vi "sInitialization.vi"(8 "UTC format":bool=TRUE, 9 "XOFF Character":u8=19 format="%.0x", 10 "XON Character":u8=17 format="%.0x", 11 "VISA resource name":refnum<visa-resource-name>="COM5") -> (0 "error IO":errorcluster, 3 "VISA resource name out":refnum<visa-resource-name>, 5 "Slow Cluster":T1)   [LabVIEW 2012]
uses:
  <vilib>/Instr/_visa.llb/VISA Configure Serial Port (Instr).vi
panel:
  out "Datanames":string[](array[string])
  out "Description":string[](array[string])
  out "Up bound":i32[](array[numeric])
  out "Low bound":i32[](array[numeric])
  out "Stopped":bool
  out "array of datanames":string[](array[string])
  out "array of datanames 2":string[](array[string])
  out "Arduino needs to be reinitialized":bool
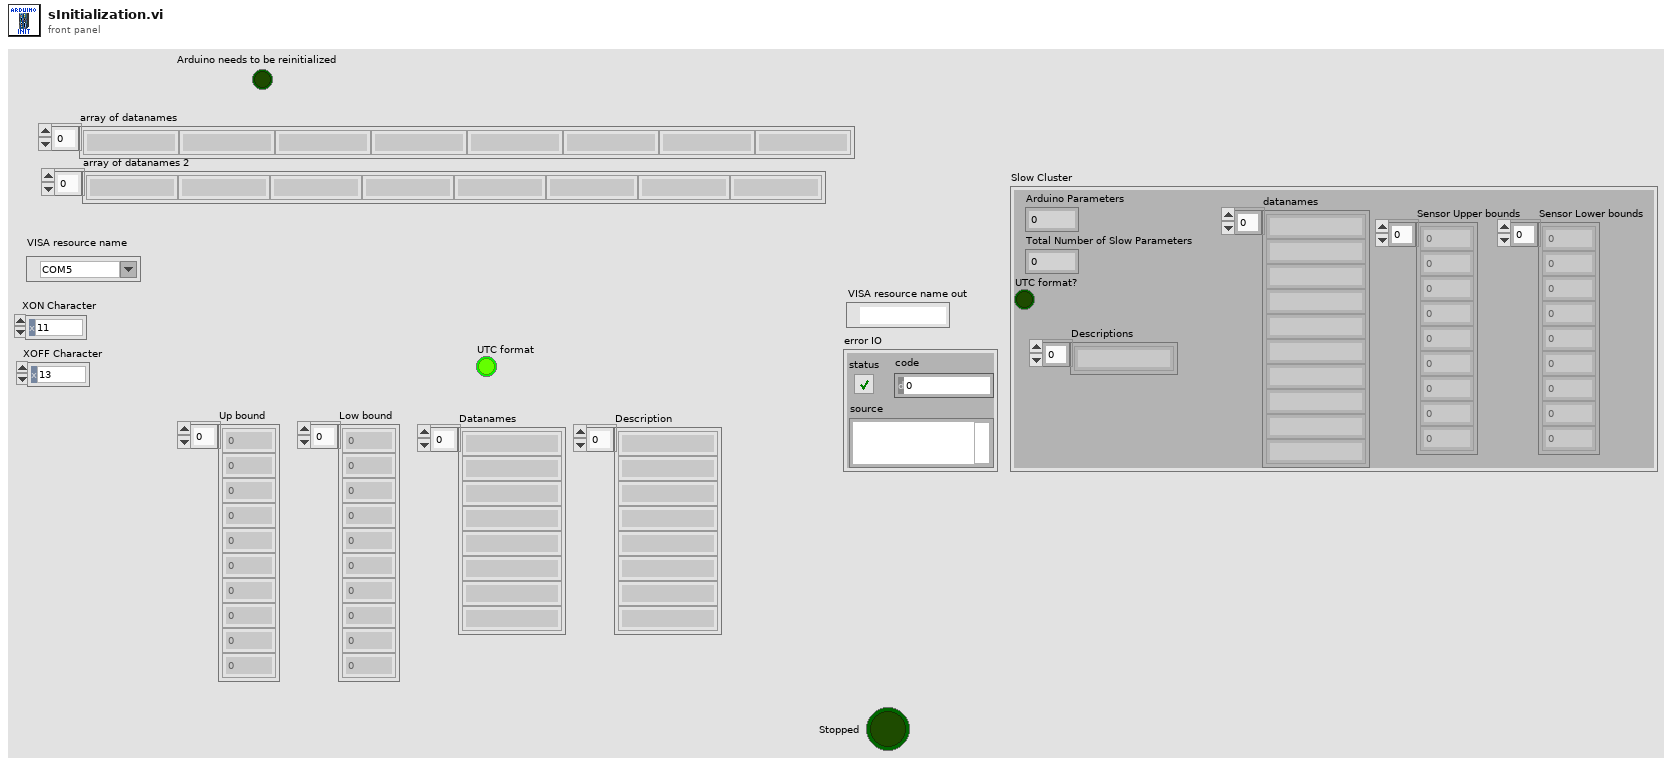
[diagram p1: front panel]
types:
  T1 = cluster{"Arduino Parameters":dbl, "Total Number of Slow Parameters":i32, "UTC format?":bool, "Sensor Upper bounds":i32[], "Sensor Lower bounds":i32[], "Descriptions":string[], "datanames":string[]}
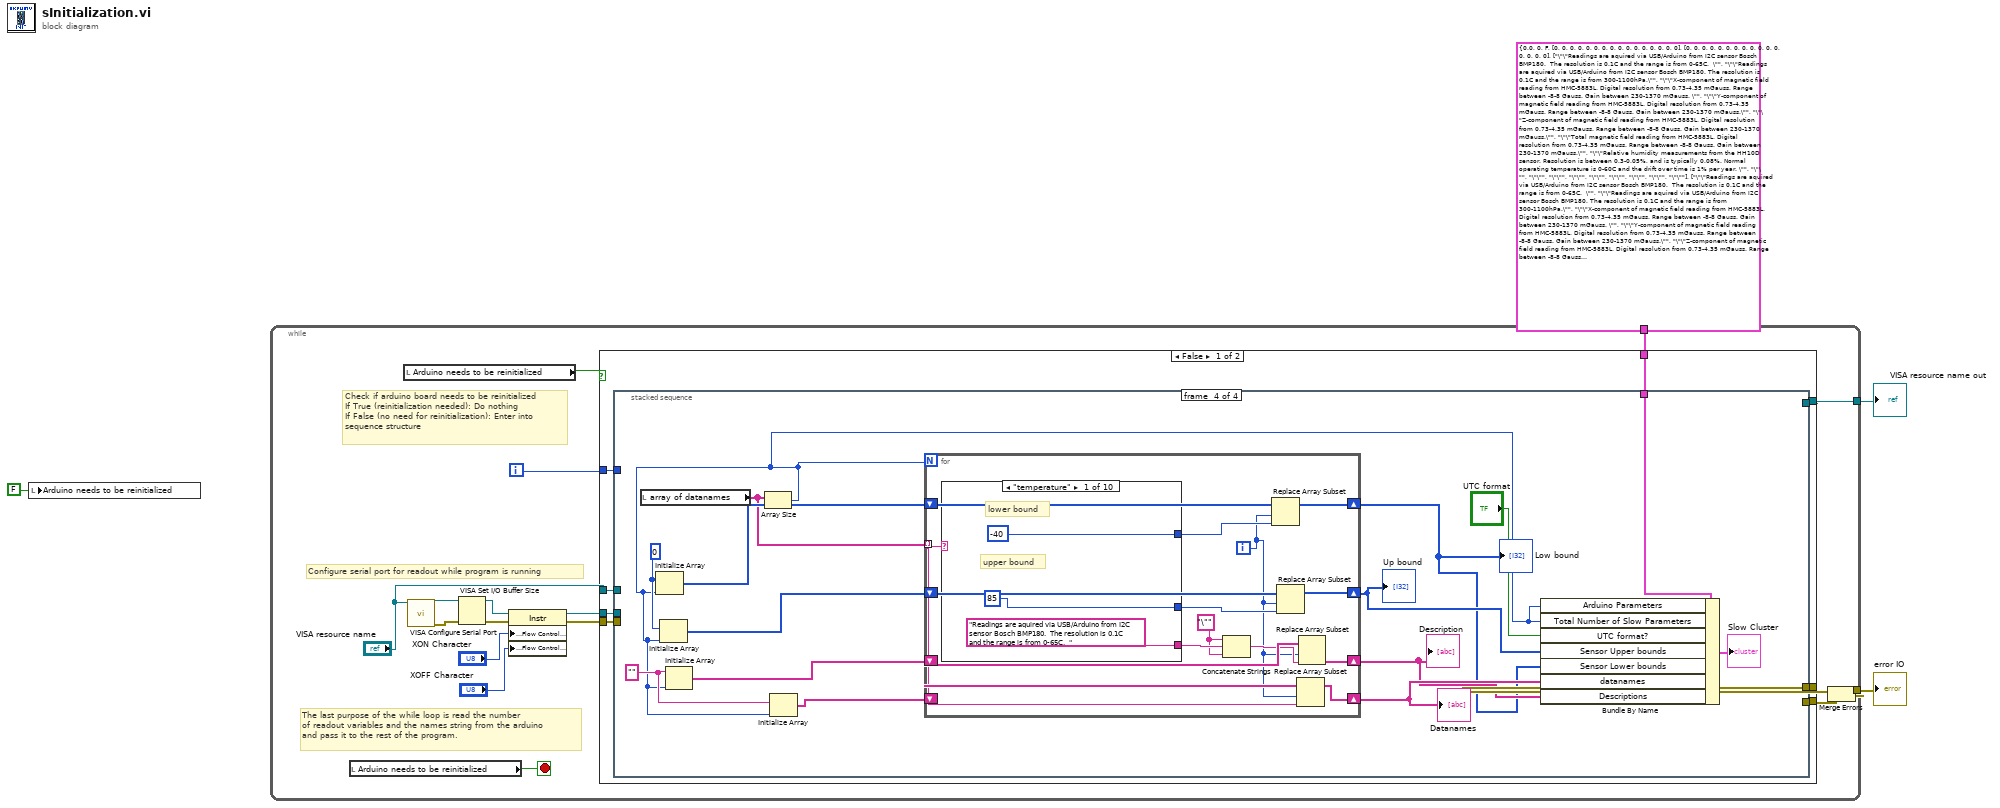
[diagram p0: block diagram]
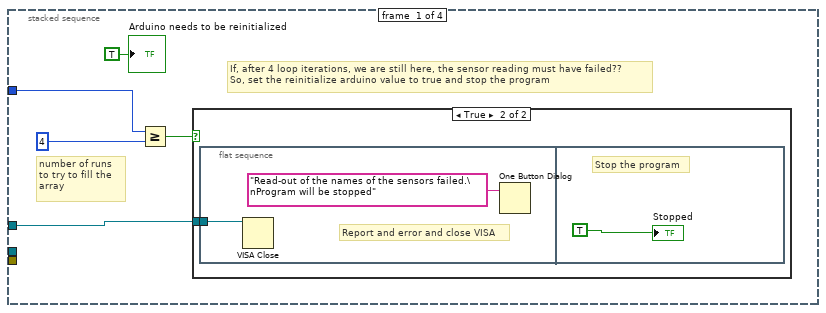
[diagram p2: hidden frame]
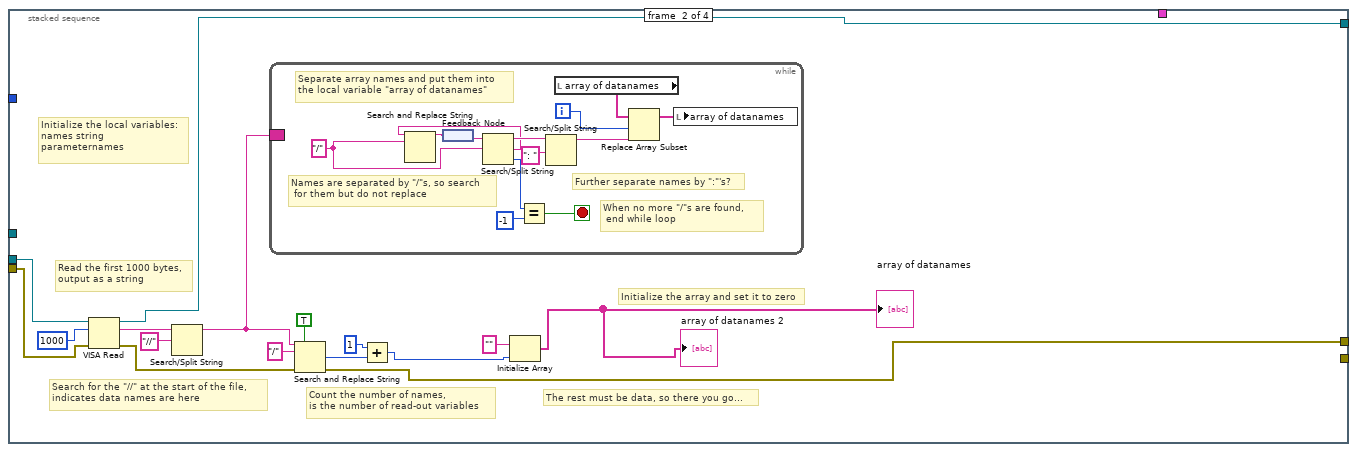
[diagram p4: hidden frame]
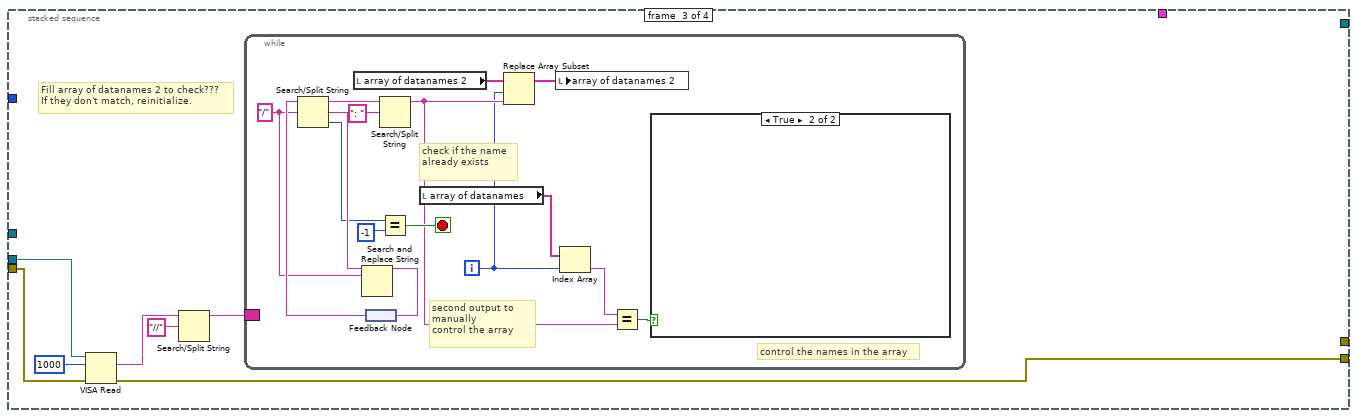
[diagram p5: hidden frame]
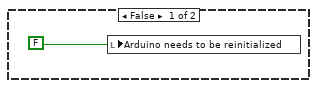
[diagram p6: hidden frame]
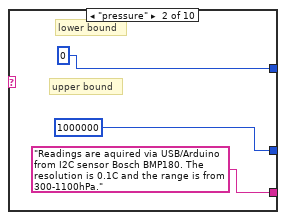
[diagram p7: hidden frame]
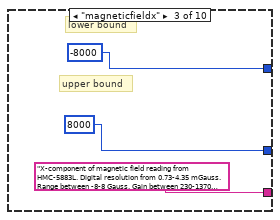
[diagram p8: hidden frame]
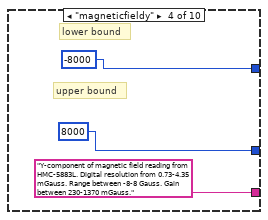
[diagram p9: hidden frame]
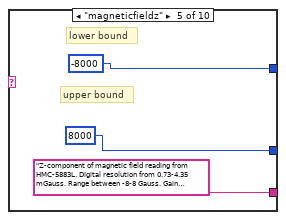
[diagram p10: hidden frame]
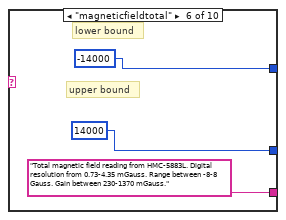
[diagram p11: hidden frame]
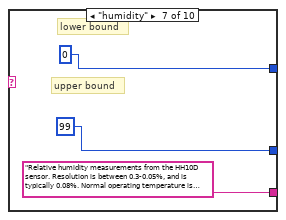
[diagram p12: hidden frame]
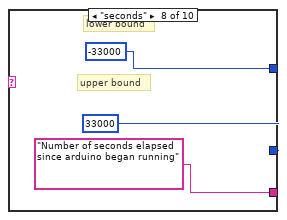
[diagram p13: hidden frame]
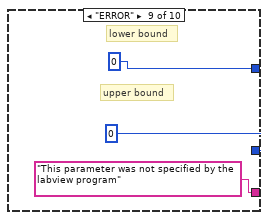
[diagram p14: hidden frame]
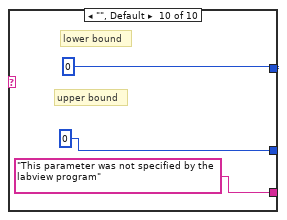
[diagram p15: hidden frame]
diagram:
  n1 = local write "Arduino needs to be reinitialized"(FALSE ("Arduino needs to be reinitialized")) -> ()
  n2 = while {
    tunnel: [w15] -> w4
    tunnel: [w14] -> w3
    tunnel: T1 {"Arduino Parameters"=0.0, "Total Number of Slow Parameters"=0, "UTC format?"=FALSE, "Sensor Upper bounds"=[0, 0, 0, 0, 0, 0, 0, 0, 0, 0, 0, 0, 0, 0, 0, 0], "Sensor Lower bounds"=[0, 0, 0, 0, 0, 0, 0, 0, 0, 0, 0, 0, 0, 0, 0, 0], "Descriptions"=["\"\"Readings are aquired via USB/Arduino from I2C sensor Bosch BMP180.  The resolution is 0.1C and the range is from 0-65C.  \"", "\"\"Readings are aquired via USB/Arduino from I2C sensor Bosch BMP180. The resolution is 0.1C and the range is from 300-1100hPa.\"", "\"\"X-component of magnetic field reading from HMC-5883L. Digital resolution from 0.73-4.35 mGauss. Range between -8-8 Gauss. Gain between 230-1370 mGauss. \"", "\"\"Y-component of magnetic field reading from HMC-5883L. Digital resolution from 0.73-4.35 mGauss. Range between -8-8 Gauss. Gain between 230-1370 mGauss.\"", "\"\"Z-component of magnetic field reading from HMC-5883L. Digital resolution from 0.73-4.35 mGauss. Range between -8-8 Gauss. Gain between 230-1370 mGauss.\"", "\"\"Total magnetic field reading from HMC-5883L. Digital resolution from 0.73-4.35 mGauss. Range between -8-8 Gauss. Gain between 230-1370 mGauss.\"", "\"\"Relative humidity measurements from the HH10D sensor. Resolution is between 0.3-0.05%, and is typically 0.08%. Normal operating temperature is 0-60C and the drift over time is 1% per year. \"", "\"\"", "\"\"", "\"\"", "\"\"", "\"\"", "\"\"", "\"\"", "\"\"", "\"\""], "datanames"=["\"\"Readings are aquired via USB/Arduino from I2C sensor Bosch BMP180.  The resolution is 0.1C and the range is from 0-65C.  \"", "\"\"Readings are aquired via USB/Arduino from I2C sensor Bosch BMP180. The resolution is 0.1C and the range is from 300-1100hPa.\"", "\"\"X-component of magnetic field reading from HMC-5883L. Digital resolution from 0.73-4.35 mGauss. Range between -8-8 Gauss. Gain between 230-1370 mGauss. \"", "\"\"Y-component of magnetic field reading from HMC-5883L. Digital resolution from 0.73-4.35 mGauss. Range between -8-8 Gauss. Gain between 230-1370 mGauss.\"", "\"\"Z-component of magnetic field reading from HMC-5883L. Digital resolution from 0.73-4.35 mGauss. Range between -8-8 Gauss. Gain between 230-1370 mGauss.\"", "\"\"Total magnetic field reading from HMC-5883L. Digital resolution from 0.73-4.35 mGauss. Range between -8-8 Gauss. Gain between 230-1370 mGauss.\"", "\"\"Relative humidity measurements from the HH10D sensor. Resolution is between 0.3-0.05%, and is typically 0.08%. Normal operating temperature is 0-60C and the drift over time is 1% per year. \"", "\"\"", "\"\"", "\"\"", "\"\"", "\"\"", "\"\"", "\"\"", "\"\"", "\"\""]} ("Cluster") -> [w5]
    i -> [w12]
    stop <- w10 stop-if-true
    # "The last purpose of the while loop is read the number \nof readout variables and the names string from the arduino\nand pass it to the rest of the program."
    # "Check if arduino board needs to be reinitialized\nIf True (reinitialization needed): Do nothing\nIf False (no need for reinitialization): Enter into \nsequence structure"
    # "Configure serial port for readout while program is running"
    n3 = local read "Arduino needs to be reinitialized"() -> (w10:bool)
    n4 = local read "Arduino needs to be reinitialized"() -> (w9:bool)
    n5 = call-poly "VISA Configure Serial Port"("VISA resource name"="VISA resource name") -> ("VISA resource name out"=w17:refnum<visa-resource-name>, "error out"=w16:errorcluster)  [unwired: 9 in, 4 out]
    n6 = VISA Set I/O Buffer Size(VISA resource name=w17, error in (no error)=w16) -> (VISA resource name out=w21:refnum<visa-resource-name>, error out=w20:errorcluster)  [unwired: 2 in]
    n7 = property class="Instr"(reference=w21, error in=w20, "Serial Settings:Flow Control XON Character"="XON Character", "Serial Settings:Flow Control XOFF Character"="XOFF Character") -> (reference out=w13:refnum<visa-resource-name>, error out=w8:errorcluster)
    n8 = case shown="False" w9 {
      tunnel: [w29 w152] -> w15
      tunnel: w13 -> [w28 w152]
      tunnel: w12 -> [w27 _]
      tunnel: "VISA resource name" -> [w26 _]
      tunnel: w8 -> [w25 _]
      tunnel: [w24 _] -> w7
      tunnel: [w23 _] -> w6
      tunnel: w5 -> [w22 _]
      frame False {
        n9 = stacked-sequence {
          tunnel: [_ w51 _ _] -> w29
          tunnel: w28 -> [_ w54 w71 _]
          tunnel: w27 -> [w34 _ _ _]
          tunnel: w26 -> [w31 _ _ _]
          tunnel: w25 -> [_ w52 w69 _]
          tunnel: [_ w41 _ _] -> w24
          tunnel: [_ _ w68 _] -> w23
          tunnel: w22 -> [_ _ _ w93]
          frame #0 {
            # "If, after 4 loop iterations, we are still here, the sensor reading must have failed??  \nSo, set the reinitialize arduino value to true and stop the program"
            # "number of runs to try to fill the array"
            n10 = Greater Or Equal?(x=w34, y=4) -> (x >= y?=w32:bool)
            n11 = case shown="True" w32 {
              tunnel: w31 -> [_ w35]
              frame False {
              }
              frame True {
                n12 = flat-sequence {
                  tunnel: w35 -> [w36]
                  frame #0 {
                    # "Report and error and close VISA"
                    n13 = VISA Close(VISA resource name=w36) -> ()  [unwired: 1 in, 1 out]
                    n14 = One Button Dialog(message="Read-out of the names of the sensors failed.\nProgram will be stopped") -> ()  [unwired: 1 in, 1 out]
                  }
                  frame #1 {
                    # "Stop the program"
                    "Stopped" <- TRUE ("stop? (T)")
                  }
                }
              }
            }
            "Arduino needs to be reinitialized" <- TRUE ("Arduino needs to be reinitialized")
          }
          frame #1 {
            # "The rest must be data, so there you go..."
            # "Count the number of names, \nis the number of read-out variables"
            # "Search for the \"//\" at the start of the file, \nindicates data names are here"
            # "Initialize the local variables: \nnames string\nparameternames"
            # "Read the first 1000 bytes, \noutput as a string"
            # "Initialize the array and set it to zero"
            n15 = VISA Read(VISA resource name=w54, byte count=u32 1000, error in (no error)=w52) -> (VISA resource name out=w51:refnum<visa-resource-name>, read buffer=w50:string, error out=w42:errorcluster)  [unwired: 1 out]
            n16 = Search/Split String(string=w50, search string/char (-)="//") -> (substring before match=w46:string)  [unwired: 1 in, 2 out]
            n17 = while {
              border: w46 -> [_]
              i -> [w55]
              stop <- w64 stop-if-true
              w60 = "/" ("search string/char (-)")
              # "Further separate names by \":\"'s?"
              # "When no more \"/\"s are found,\n end while loop"
              # "Names are separated by \"/\"s, so search\n for them but do not replace"
              # "Separate array names and put them into \nthe local variable \"array of datanames\""
              n18 = feedback #1() -> (w62:string)
              n19 = Search/Split String(string=w62, search string/char (-)=w60) -> (substring before match=w58:string, match + rest of string=w57:string, offset of match=w59:i32)  [unwired: 1 in]
              n20 = Search and Replace String(input string=w57, search string=w60) -> (result string=w61:string)  [unwired: 6 in, 3 out]
              n21 = feedback-in #1(w61) -> ()
              n22 = Equal?(x=w59, y=-1) -> (x = y?=w64:bool)
              n23 = Search/Split String(string=w58, search string/char (-)=": " ("format string")) -> (substring before match=w56:string)  [unwired: 1 in, 2 out]
              n24 = local read "array of datanames"() -> (w66:string[])
              n25 = Replace Array Subset(array=w66, new element=w56, index=w55) -> (w65:string[])
              n26 = local write "array of datanames"(w65) -> ()
            }
            n27 = Search and Replace String(replace all?=TRUE ("replace all? (F)"), input string=w46, search string="/", error in=w42) -> (number of replacements=w47:i32, error out=w41:errorcluster)  [unwired: 4 in, 2 out]
            n28 = Add(x=1, y=w47) -> (x+y=w39:i32)
            n29 = Initialize Array("", w39) -> (→"array of datanames" →"array of datanames 2":string[])
          }
          frame #2 {
            # "Fill array of datanames 2 to check???\nIf they don't match, reinitialize."
            n30 = VISA Read(VISA resource name=w71, byte count=u32 1000, error in (no error)=w69) -> (read buffer=w74:string, error out=w68:errorcluster)  [unwired: 2 out]
            n31 = Search/Split String(string=w74, search string/char (-)="//") -> (substring before match=w70:string)  [unwired: 1 in, 2 out]
            n32 = while {
              border: w70 -> [_]
              i -> [w75]
              stop <- w86 stop-if-true
              w81 = "/" ("search string/char (-)")
              # "second output to manually\ncontrol the array"
              # "check if the name already exists"
              # "control the names in the array"
              n33 = local read "array of datanames 2"() -> (w88:string[])
              n34 = feedback #2() -> (w84:string)
              n35 = Search/Split String(string=w84, search string/char (-)=w81) -> (substring before match=w89:string, match + rest of string=w83:string, offset of match=w80:i32)  [unwired: 1 in]
              n36 = Search and Replace String(input string=w83, search string=w81) -> (result string=w82:string)  [unwired: 6 in, 3 out]
              n37 = feedback-in #2(w82) -> ()
              n38 = Search/Split String(string=w89, search string/char (-)=": " ("format string")) -> (substring before match=w77:string)  [unwired: 1 in, 2 out]
              n39 = Equal?(x=w80, y=-1) -> (x = y?=w86:bool)
              n40 = local read "array of datanames"() -> (w78:string[])
              n41 = Replace Array Subset(array=w88, new element=w77, index=w75) -> (w87:string[])
              n42 = local write "array of datanames 2"(w87) -> ()
              n43 = Index Array(array=w78, index=w75) -> (element=w79:string)
              n44 = Equal?(x=w79, y=w77) -> (x = y?=w76:bool)
              n45 = case shown="True" w76 {
                frame False {
                  n46 = local write "Arduino needs to be reinitialized"(FALSE ("reinitialize arduino read boolean")) -> ()
                }
                frame True {
                }
              }
            }
          }
          frame #3 {
            w100 = ""
            w106 = 0 ("element")
            n47 = local read "array of datanames"() -> (w101:string[])
            n48 = Array Size(array=w101) -> (size(s)=w94:i32)
            n49 = Initialize Array(w106, w94) -> (w105:i32[])
            n50 = Initialize Array(w106, w94) -> (w104:i32[])
            n51 = Initialize Array(w100, w94) -> (w103:string[])
            n52 = Initialize Array(w100, w94) -> (w102:string[])
            n53 = for {
              N: w94 -> [_]
              tunnel: w101 -> [w107] mode=indexing
              shift-right: [w116] -> w97
              shift-left: w104 -> [w120]
              shift-right: [w117] -> w96
              shift-left: w105 -> [w121]
              shift-right: [w114] -> w98
              shift-left: w103 -> [w115]
              shift-right: [w108] -> w99
              shift-left: w102 -> [w110]
              i -> [w109]
              w112 = "\"" ("string")
              n54 = case shown="\"temperature\"" w107 {
                tunnel: [85 1000000 8000 8000 8000 14000 99 33000 0 0] -> w118
                tunnel: [-40 0 -8000 -8000 -8000 -14000 0 -33000 0 0] -> w119
                tunnel: ["Readings are aquired via USB/Arduino from I2C sensor Bosch BMP180.  The resolution is 0.1C and the range is from 0-65C.  " ("XML Tag") "Readings are aquired via USB/Arduino from I2C sensor Bosch BMP180. The resolution is 0.1C and the range is from 300-1100hPa." "X-component of magnetic field reading from HMC-5883L. Digital resolution from 0.73-4.35 mGauss. Range between -8-8 Gauss. Gain between 230-1370 mGauss. " "Y-component of magnetic field reading from HMC-5883L. Digital resolution from 0.73-4.35 mGauss. Range between -8-8 Gauss. Gain between 230-1370 mGauss." "Z-component of magnetic field reading from HMC-5883L. Digital resolution from 0.73-4.35 mGauss. Range between -8-8 Gauss. Gain between 230-1370 mGauss." "Total magnetic field reading from HMC-5883L. Digital resolution from 0.73-4.35 mGauss. Range between -8-8 Gauss. Gain between 230-1370 mGauss." "Relative humidity measurements from the HH10D sensor. Resolution is between 0.3-0.05%, and is typically 0.08%. Normal operating temperature is 0-60C and the drift over time is 1% per year. " "Number of seconds elapsed since arduino began running" ("XML Tag") "This parameter was not specified by the labview program" ("XML Tag") "This parameter was not specified by the labview program" ("XML Tag")] -> w113
                frame "temperature" {
                  # "upper bound"
                  # "lower bound"
                }
                frame "pressure" {
                  # "upper bound"
                  # "lower bound"
                }
                frame "magneticfieldx" {
                  # "upper bound"
                  # "lower bound"
                }
                frame "magneticfieldy" {
                  # "upper bound"
                  # "lower bound"
                }
                frame "magneticfieldz" {
                  # "upper bound"
                  # "lower bound"
                }
                frame "magneticfieldtotal" {
                  # "upper bound"
                  # "lower bound"
                }
                frame "humidity" {
                  # "upper bound"
                  # "lower bound"
                }
                frame "seconds" {
                  # "upper bound"
                  # "lower bound"
                }
                frame "ERROR" {
                  # "upper bound"
                  # "lower bound"
                }
                frame "", Default {
                  # "upper bound"
                  # "lower bound"
                }
              }
              n55 = Concatenate Strings(w112, w113, w112) -> (w111:string)
              n56 = Replace Array Subset(array=w121, new element=w119, index=w109) -> (w117:i32[])
              n57 = Replace Array Subset(array=w120, new element=w118, index=w109) -> (w116:i32[])
              n58 = Replace Array Subset(array=w110, new element=w107, index=w109) -> (w108:string[])
              n59 = Replace Array Subset(array=w115, new element=w111, index=w109) -> (w114:string[])
            }
            "Low bound" <- w96
            "Up bound" <- w97
            "Description" <- w98
            "Datanames" <- w99
            n60 = Bundle By Name(cluster=w93, "Arduino Parameters"=w94, "Total Number of Slow Parameters"=w94, "UTC format?"="UTC format", "Sensor Upper bounds"=w97, "Sensor Lower bounds"=w96, "datanames"=w99, "Descriptions"=w98) -> (→"Slow Cluster":T1)
          }
        }
      }
      frame True {
      }
    }
    n61 = Merge Errors(w7, w6) -> (w14:errorcluster)
  }
  "VISA resource name out" <- w4
  "error IO" <- w3
